vi "KV_VolHead_Addr_Reset.vi"() -> (3 "OK?":bool)   [LabVIEW 2015]
uses:
  <vilib>/Instr/_visa.llb/VISA Configure Serial Port (Instr).vi
panel:
  in  "MyIndex":u8
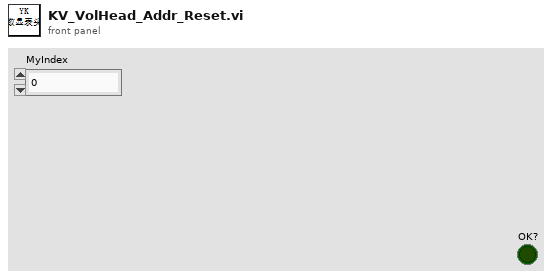
[diagram p1: front panel]
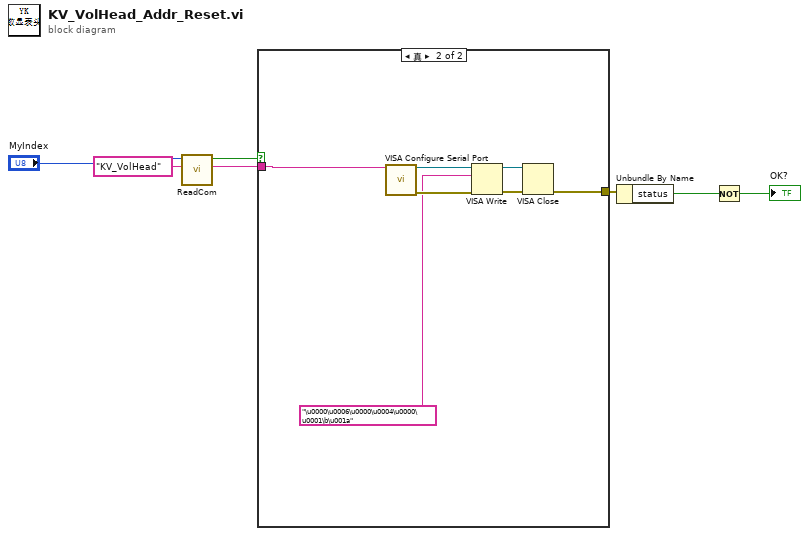
[diagram p0: block diagram]
diagram:
  n1 = call "ReadCom.vi"("仪器名称"="KV_VolHead", "MyIndex"="MyIndex") -> ("COM"=w1:string, "OK?"=w2:bool)  [unwired: 7 in, 1 out]
  n2 = case shown="真" w2 {
    tunnel: [_ w9] -> w7
    tunnel: w1 -> [_ w10]
    frame False {
    }
    frame True {
      n3 = call-poly "VISA Configure Serial Port"("VISA resource name"=w10) -> ("VISA resource name out"=w14:refnum<visa-resource-name>, "error out"=w13:errorcluster)  [unwired: 13 in]
      n4 = VISA Write(VISA resource name=w14, write buffer="\u0000\u0006\u0000\u0004\u0000\u0001\b\u001a", error in (no error)=w13) -> (VISA resource name out=w8:refnum<visa-resource-name>, error out=w11:errorcluster)  [unwired: 1 out]
      n5 = VISA Close(VISA resource name=w8, error in (no error)=w11) -> (error out=w9:errorcluster)
    }
  }
  n6 = Unbundle By Name(w7) -> ("status"=w6:bool)
  n7 = Not(x=w6) -> (.not. x?=→"OK?":bool)
